vi "Draw_Sources.vi"(6 "address in":string, 8 "error in (no error)":errorcluster, 9 "disable contained items?":bool, 10 "Source in":refnum<class "IB_Source.lvclass">[](array[class]), 11 "IB_DestTree in":refnum<class "IB_Tree_Dest.lvclass">) -> (0 "error out":errorcluster, 3 "source":refnum<class "IB_Tree_Item_Source.lvclass">[](array[class]))   [LabVIEW 2020, in "IB_Tree_Dest.lvclass"]
uses:
  <vilib>/AppBuilder/IB_Classes/Tree_Dest/IB_Tree_Dest.lvclass
  <vilib>/AppBuilder/IB_Classes/Tree_Dest/IB_Tree_Dest.lvclass/IB_Tree_Dest.ctl
  <vilib>/AppBuilder/IB_Classes/Tree/IB_Tree.lvclass
  <vilib>/AppBuilder/IB_Classes/Source/IB_Source.lvclass
  <vilib>/AppBuilder/IB_Classes/Tree_Item_Source/IB_Tree_Item_Source.lvclass
  e:/builds/penguin/labview/branches/2020/dev/dist/vi.lib/AppBuilder/IB_Classes/Tree/IB_Tree.lvclass
  e:/builds/penguin/labview/branches/2020/dev/dist/vi.lib/AppBuilder/IB_Classes/Tree_Dest/IB_Tree_Dest.lvclass
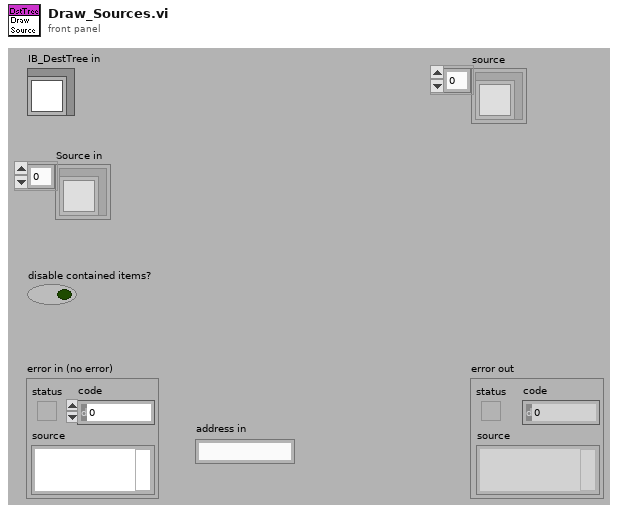
[diagram p1: front panel]
types:
  T1 = typedef "IB_Source.ctl" = cluster{"name":string, "sourceTag":string, "destTag":string, "path":path, "eng_installPath":string, "UI_inBuild?":bool, "str ref?":bool}
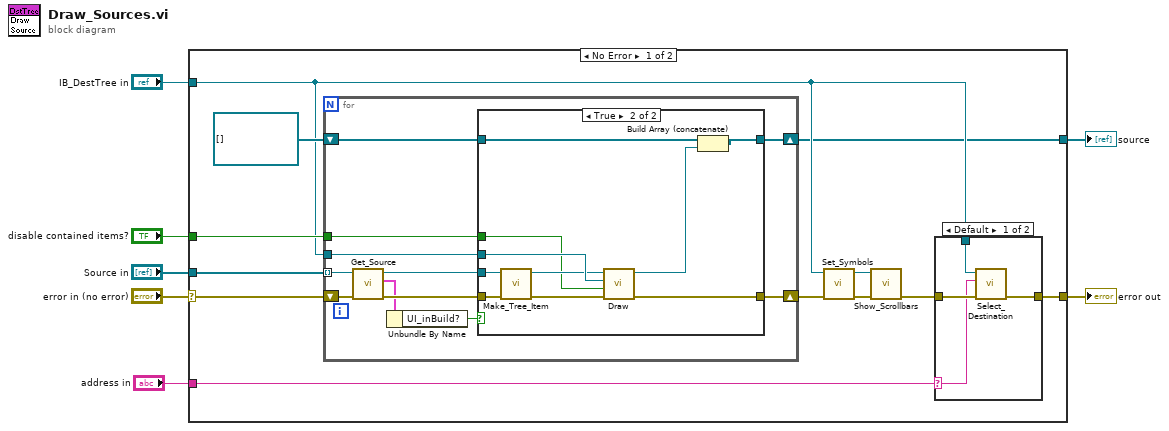
[diagram p0: block diagram]
diagram:
  n1 = case shown="No Error" "error in (no error)" {
    selector: "error in (no error)" -> [w18 w48]
    tunnel: [w10 w48] -> w6
    tunnel: "IB_DestTree in" -> [w12 _]
    tunnel: "Source in" -> [w19 _]
    tunnel: [w9 _] -> w3
    tunnel: "disable contained items?" -> [w13 _]
    tunnel: "address in" -> [w8 _]
    frame No Error {
      n2 = for {
        tunnel: w19 -> [w30] mode=indexing
        shift-right: [w35] -> w17
        shift-left: w18 -> [w28]
        tunnel: w12 -> [w34]
        shift-right: [w32] -> w9
        shift-left: refnum<class "IB_Tree_Item_Source.lvclass">[] [] -> [w33]
        tunnel: w13 -> [w31]
        n3 = call <vilib>:"Get_Source.vi"("error in (no error)"=w28, "IB_Source in"=w30) -> ("error out"=w27:errorcluster, "data"=w26:T1, "IB_Source out"=w29:refnum<class "IB_Source.lvclass">)  [unwired: 7 out]
        n4 = Unbundle By Name(w26) -> ("UI_inBuild?"=w25:bool)
        n5 = case shown="True" w25 {
          tunnel: w27 -> [w36 w47]
          tunnel: [w36 w46] -> w35
          tunnel: w29 -> [_ w45]
          tunnel: w34 -> [_ w43]
          tunnel: w33 -> [w37 w41]
          tunnel: [w37 w40] -> w32
          tunnel: w31 -> [_ w39]
          frame False {
          }
          frame True {
            n6 = call-dynamic "Make_Tree_Item.vi"("error in (no error)"=w47, "IB_Source in"=w45) -> ("error out"=w44:errorcluster, "TreeSrcItem"=w42:refnum<class "IB_Tree_Item_Source.lvclass">)  [unwired: 1 in, 7 out]
            n7 = call-dynamic "Draw.vi"("error in (no error)"=w44, "disable contained items?"=w39, "IB_Tree"=w43, "IB_TreeItem in"=w42) -> ("error out"=w46:errorcluster, "IB_TreeItem out"=w38:refnum<class "IB_Tree_Item_Source.lvclass">)  [unwired: 6 out]
            n8 = Build Array (concatenate)(w41, w38) -> (w40:refnum<class "IB_Tree_Item_Source.lvclass">[])
          }
        }
      }
      n9 = call <vilib>:"Set_Symbols.vi"("error in (no error)"=w17, "IB_Tree in"=w12) -> ("error out"=w15:errorcluster, "IB_Tree out"=w16:refnum<class "IB_Tree_Dest.lvclass">)  [unwired: 8 out]
      n10 = call <vilib>:"Show_Scrollbars.vi"("error in (no error)"=w15, "IB_Tree in"=w16) -> ("error out"=w11:errorcluster)  [unwired: 9 out]
      n11 = case shown="Default" w8 {
        selector: w8 -> [w20 _]
        tunnel: w12 -> [w23 _]
        tunnel: w11 -> [w22 w24]
        tunnel: [w21 w24] -> w10
        frame Default {
          n12 = call <vilib>:"Select_Destination.vi"("error in (no error)"=w22, "destTag"=w20, "IB_DestTree in"=w23) -> ("error out"=w21:errorcluster)  [unwired: 8 out]
        }
        frame "" {
        }
      }
    }
    frame Error {
    }
  }
  "error out" <- w6
  "source" <- w3
